vi "Find Tag.vi"(3 "string":string, 4 "close tag":string, 5 "open tag":string) -> (0 "Length":i32[](array[numeric]), 1 "Start":i32[](array[numeric]), 2 "string out":string)   [LabVIEW 2018]
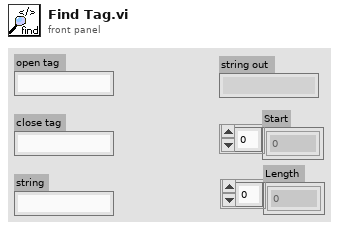
[diagram p1: front panel]
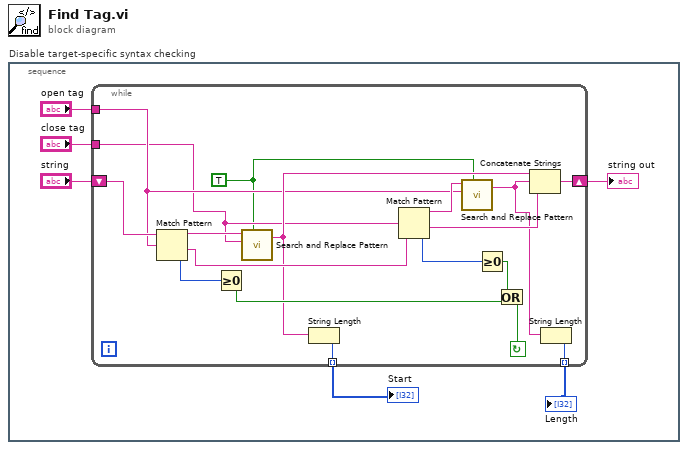
[diagram p0: block diagram]
diagram:
  n1 = stacked-sequence "Disable target-specific syntax checking" {
    frame #0 {
      n2 = while {
        tunnel: [w24] -> w1 mode=indexing
        tunnel: [w23] -> w2 mode=indexing
        shift-right: [w19] -> w4
        shift-left: "string" -> [w21]
        tunnel: "open tag" -> [w9]
        tunnel: "close tag" -> [w8]
        stop <- w14 continue-if-true
        w7 = TRUE ("replace all? (F)")
        n3 = Match Pattern(string=w21, regular expression=w9) -> (before substring=w11:string, after substring=w22:string, offset past match=w18:i32)  [unwired: 1 in, 1 out]
        n4 = Greater Or Equal To 0?(x=w18) -> (x >= 0?=w15:bool)
        n5 = call "Search and Replace Pattern.vi"("string"=w11, "regular expression (\"\")"=w8, "replace all? (F)"=w7) -> ("result string"=w10:string)  [unwired: 2 in, 1 out]
        n6 = String Length(string=w10) -> (length=w24:i32)
        n7 = Match Pattern(string=w22, regular expression=w8) -> (before substring=w13:string, after substring=w20:string, offset past match=w17:i32)  [unwired: 1 in, 1 out]
        n8 = call "Search and Replace Pattern.vi"("string"=w13, "regular expression (\"\")"=w9, "replace all? (F)"=w7) -> ("result string"=w12:string)  [unwired: 2 in, 1 out]
        n9 = Greater Or Equal To 0?(x=w17) -> (x >= 0?=w16:bool)
        n10 = Or(x=w16, y=w15) -> (x .or. y?=w14:bool)
        n11 = Concatenate Strings(w10, w12, w20) -> (w19:string)
        n12 = String Length(string=w12) -> (length=w23:i32)
      }
      "string out" <- w4
      "Length" <- w2
      "Start" <- w1
    }
  }
